vi "Refresh Online CSMs in lvcsm.vi"(7 "Caller":string, 8 "Error In":errorcluster caption="error in (no error)") -> (0 "error out":errorcluster, 1 "Array W/ Subset Deleted":string[](array[string]))   [LabVIEW 2017, in "CSM-Helper API with lvcsm Support.lvlib"]
uses:
  CSM-Helper API with lvcsm Support.lvlib
  Communicable State Machine.lvlib
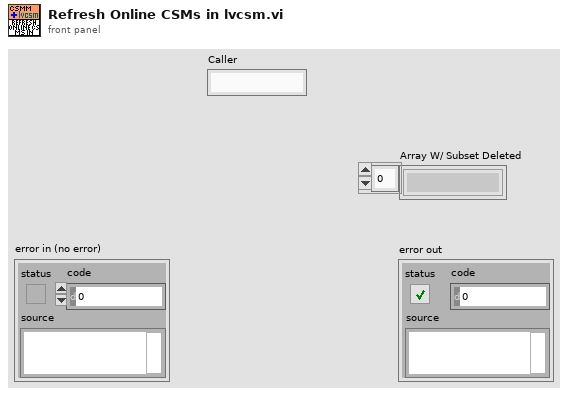
[diagram p1: front panel]
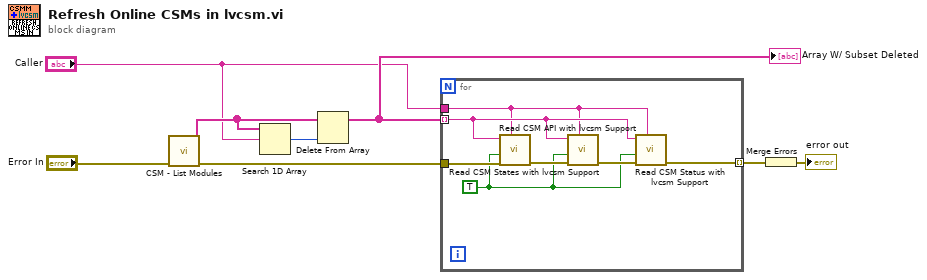
[diagram p0: block diagram]
diagram:
  n1 = call "CSM - List Modules.vi"("Error In"="Error In") -> ("error out"=w8:errorcluster, "Module Names"=w5:string[])  [unwired: 9 in]
  n2 = Search 1D Array(1D array=w5, element="Caller") -> (index of element=w3:i32)  [unwired: 1 in]
  n3 = Delete From Array(array=w5, index=w3) -> (array with subset deleted=w6:string[])  [unwired: 1 in, 1 out]
  "Array W/ Subset Deleted" <- w6
  n4 = for {
    tunnel: w8 -> [w15]
    tunnel: w6 -> [w11] mode=indexing
    tunnel: "Caller" -> [w10]
    tunnel: [w12] -> w7 mode=indexing
    w9 = TRUE ("Force?(F)")
    n5 = call "Read CSM API with lvcsm Support.vi"("Current Module (\"\" to Generate an ID)"=w10, "error in (no error)"=w15, "Force? (F)"=w9, "CSM Name"=w11) -> ("error out"=w14:errorcluster)  [unwired: 6 in, 1 out]
    n6 = call "Read CSM States with lvcsm Support.vi"("Current Module (\"\" to Generate an ID)"=w10, "error in (no error)"=w14, "Force? (F)"=w9, "CSM Name"=w11) -> ("error out"=w13:errorcluster)  [unwired: 6 in, 1 out]
    n7 = call "Read CSM Status with lvcsm Support.vi"("Current Module (\"\" to Generate an ID)"=w10, "error in (no error)"=w13, "Force? (F)"=w9, "CSM Name"=w11) -> ("error out"=w12:errorcluster)  [unwired: 6 in, 1 out]
  }
  n8 = Merge Errors(w7) -> (→"error out":errorcluster)
